vi "solar_cfg Core Desc.vi"(7 "Allow Multi-Line? (F)":bool, 10 "Key":string, 11 "Comments (Key,Comment)":cluster{"Key":string, "Comment":string}[](array[cluster])) -> (3 "Comment":string)   [LabVIEW 2018]
doc: "This VI searches for the key specified and appends the comment if found. Use '*' to append a comment for every key."
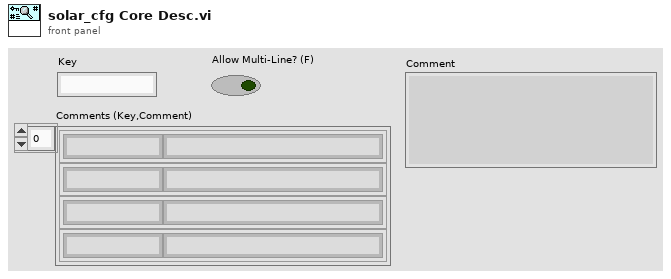
[diagram p1: front panel]
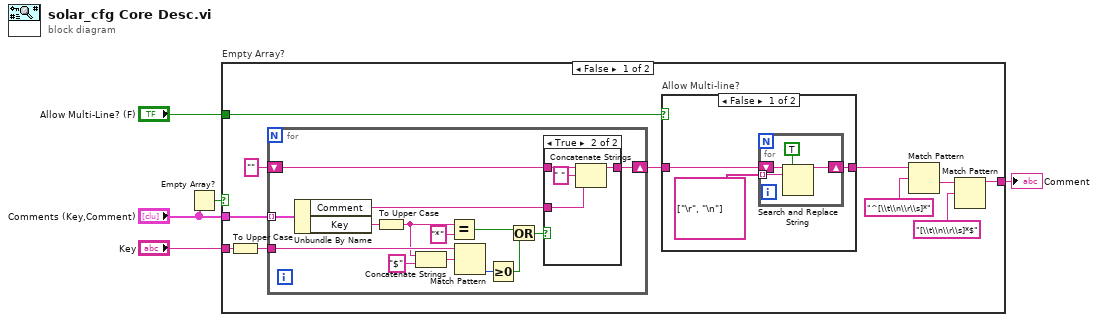
[diagram p0: block diagram]
diagram:
  n1 = Empty Array?(array="Comments (Key,Comment)") -> (empty?=w1:bool)
  n2 = case "Empty Array?" shown="False" w1 {
    tunnel: "Key" -> [w16 _]
    tunnel: "Comments (Key,Comment)" -> [w15 _]
    tunnel: "Allow Multi-Line? (F)" -> [w11 _]
    tunnel: [w10 _] -> w3
    frame False {
      n3 = To Upper Case(1:w16) -> (0:w14:string)
      n4 = for {
        tunnel: w15 -> [w19] mode=indexing
        tunnel: w14 -> [w25]
        shift-right: [w27] -> w12
        shift-left: "" -> [w26]
        n5 = Unbundle By Name(w19) -> ("Comment"=w17:string, "Key"=w18:string)
        n6 = To Upper Case(1:w18) -> (0:w24:string)
        n7 = Concatenate Strings(w24, "$" ("string")) -> (w23:string)
        n8 = Equal?(x=w24, y="*") -> (x = y?=w28:bool)
        n9 = Match Pattern(string=w25, regular expression=w23) -> (offset past match=w21:i32)  [unwired: 1 in, 3 out]
        n10 = Greater Or Equal To 0?(x=w21) -> (x >= 0?=w20:bool)
        n11 = Or(x=w28, y=w20) -> (x .or. y?=w30:bool)
        n12 = case shown="True" w30 {
          tunnel: w17 -> [_ w35]
          tunnel: [w31 w34] -> w27
          tunnel: w26 -> [w31 w33]
          frame False {
          }
          frame True {
            n13 = Concatenate Strings(w33, " " ("string"), w35) -> (w34:string)
          }
        }
      }
      n14 = case "Allow Multi-line?" shown="False" w11 {
        tunnel: w12 -> [w38 w43]
        tunnel: [w37 w43] -> w9
        frame False {
          n15 = for {
            tunnel: string[] ["\r", "\n"] -> [w39] mode=indexing
            shift-right: [w41] -> w37
            shift-left: w38 -> [w42]
            n16 = Search and Replace String(replace all?=TRUE ("replace all? (F)"), input string=w42, search string=w39) -> (result string=w41:string)  [unwired: 5 in, 3 out]
          }
        }
        frame True {
        }
      }
      n17 = Match Pattern(string=w9, regular expression="^[\\t\\n\\r\\s]*") -> (after substring=w8:string)  [unwired: 1 in, 3 out]
      n18 = Match Pattern(string=w8, regular expression="[\\t\\n\\r\\s]*$") -> (before substring=w10:string)  [unwired: 1 in, 3 out]
    }
    frame True {
    }
  }
  "Comment" <- w3
